vi "StudentScope - Timebase Convert.vi"(1 "Sec/Div":u32) -> (0 "Sec/Div":dbl)   [LabVIEW 2015]
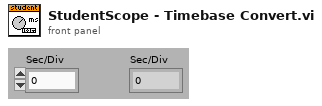
[diagram p1: front panel]
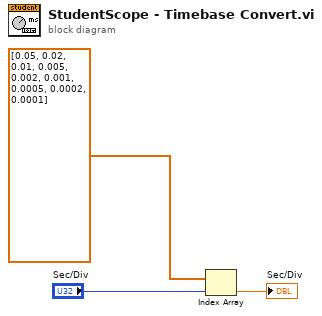
[diagram p0: block diagram]
diagram:
  n1 = Index Array(array=dbl[] [0.05, 0.02, 0.01, 0.005, 0.002, 0.001, 0.0005, 0.0002, 0.0001] ("reversed array"), index="Sec/Div") -> (element=→"Sec/Div":dbl)
